vi "Configure FFT Measurement Averaging Mode.vi"(8 "error in (no error)":errorcluster, 9 "Averaging Mode (Logarithmic)":i32(ring)=1 items=["Linear", "Logarithmic"], 10 "Instance (1)":i32=1, 11 "VISA resource name":refnum<visa-resource-name>) -> (0 "error out":errorcluster, 3 "VISA resource name out":refnum<visa-resource-name>)   [LabVIEW 2015, in "Rohde&Schwarz CMXP GPRF.lvlib"]
doc: "Selects the averaging mode for the average FFT trace.\n\nAttribute:\nRSCMXPGPRF_ATTR_FFT_MEASUREMENT_AVERAGING_MODE\n\nRemote-control command:\nCONFigure:GPRF:MEAS<i>:FFTSanalyzer:AMODe"
uses:
  <instrlib>/Rohde&Schwarz CMXP GPRF/Rohde&Schwarz CMXP GPRF.lvlib
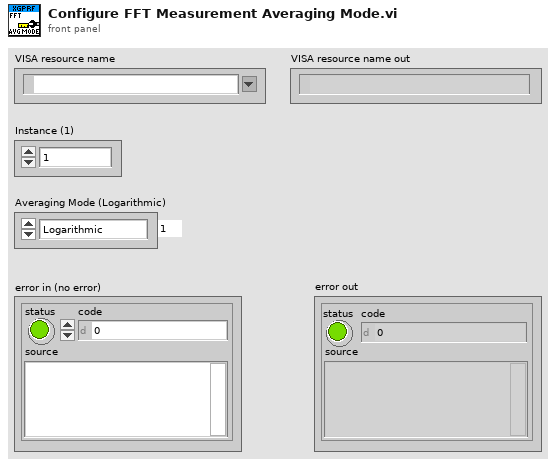
[diagram p1: front panel]
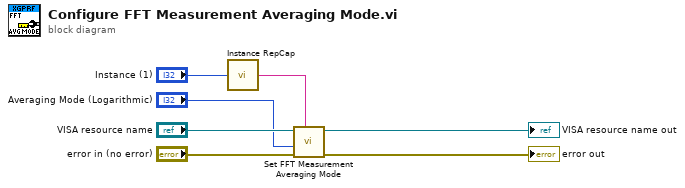
[diagram p0: block diagram]
diagram:
  n1 = call <instrlib>:"Instance RepCap.vi"("instance  in"="Instance (1)") -> ("instance out"=w7:string)
  n2 = call "Set FFT Measurement Averaging Mode"("Repeated Capabilities"=w7, "error in (no error)"="error in (no error)", "FFT Measurement Averaging Mode (0 - Linear)"="Averaging Mode (Logarithmic)", "instrument handle"="VISA resource name") -> ("error out"=→"error out":errorcluster, "instrument handle out"=→"VISA resource name out":refnum<visa-resource-name>)  [unwired: 6 in]
